vi "get channel property.vi"(8 "error in":errorcluster, 10 "property":string, 11 "channel in":refnum<class "TBM channel.lvclass">) -> (0 "error out":errorcluster, 1 "value":string, 3 "channel out":refnum<class "TBM channel.lvclass">)   [LabVIEW 2013, in "TBM channel.lvclass"]
uses:
  TBM channel.lvclass
  <vilib>/NI/Tag Bus/tag/tag descriptor.lvclass/tag descriptor.ctl
  TBM channel.lvclass/TBM channel.ctl
  <vilib>/NI/Tag Bus/tag/tag descriptor.lvclass
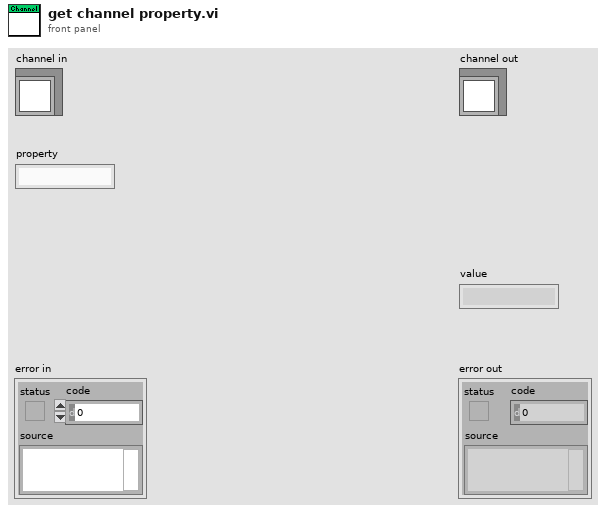
[diagram p1: front panel]
types:
  T1 = typedef "tag bus.lvlib/tag descriptor.lvclass/Data Type.ctl" = enum16{"Double", "Single", "I64", "I32", "I16", "I8", "U64", "U32", "U16", "U8", "Boolean", "String", "Array of Double", "Array of Single", "Array of I64", "Array of I32", "Array of I16", "Array of I8", "Array of U64", "Array of U32", "Array of U16", "Array of U8", "Array of Boolean", "Array of String"}
  T2 = typedef "TBM channel.lvclass/channel classification.ctl" = enum16{"input data", "output data", "processing parameter", "processing result"}
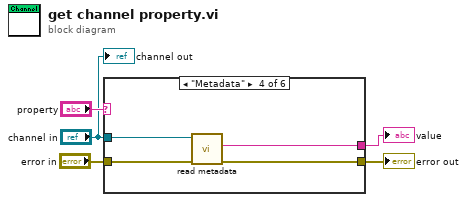
[diagram p0: block diagram]
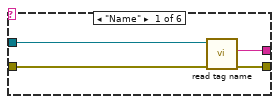
[diagram p2: hidden frame]
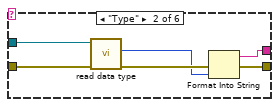
[diagram p3: hidden frame]
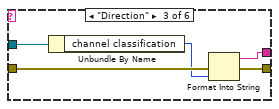
[diagram p4: hidden frame]
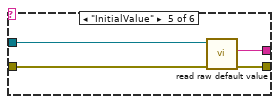
[diagram p5: hidden frame]
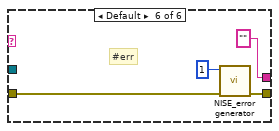
[diagram p6: hidden frame]
diagram:
  n1 = case shown="\"Metadata\"" "property" {
    tunnel: [w8 w12 w18 w23 w27 w31] -> w3
    tunnel: "error in" -> [w9 w14 w19 w24 w28 w32]
    tunnel: "channel in" -> [w7 w15 w20 w22 w26 _]
    tunnel: [w6 w10 w16 w21 w25 "" ("raw default")] -> w1
    frame "Name" {
      n2 = call <vilib>:"read tag name.vi"("error in"=w9, "system tag in"=w7) -> ("error out"=w8:errorcluster, "name"=w6:string)  [unwired: 7 in, 1 out]
    }
    frame "Type" {
      n3 = call <vilib>:"read data type.vi"("error in"=w14, "system tag in"=w15) -> ("error out"=w13:errorcluster, "data type"=w11:T1)  [unwired: 7 in, 1 out]
      n4 = Format Into String(error in=w13, w11) -> (resulting string=w10:string, error out=w12:errorcluster)  [unwired: 2 in]
    }
    frame "Direction" {
      n5 = Unbundle By Name(w20) -> ("channel classification"=w17:T2)
      n6 = Format Into String(error in=w19, w17) -> (resulting string=w16:string, error out=w18:errorcluster)  [unwired: 2 in]
    }
    frame "Metadata" {
      n7 = call <vilib>:"read metadata.vi"("error in"=w24, "system tag in"=w22) -> ("error out"=w23:errorcluster, "metadata"=w21:string)  [unwired: 7 in, 1 out]
    }
    frame "InitialValue" {
      n8 = call <vilib>:"read raw default value.vi"("error in"=w28, "system tag in"=w26) -> ("error out"=w27:errorcluster, "raw default"=w25:string)  [unwired: 7 in, 1 out]
    }
    frame Default {
      # "#err"
      n9 = call <vilib>:"NISE_error generator.vi"("error in"=w32, "error code (0)"=1) -> ("error out"=w31:errorcluster)  [unwired: 7 in]
    }
  }
  "error out" <- w3
  "value" <- w1
  "channel out" <- "channel in"
